vi "Temperature Warnings.vi"() -> ()   [LabVIEW 2018]
doc: "This VI is used to determine the string to output to the weather station based on the current temperature and limit settings.\n\nInputs: Current Temperature (DBL), Minimum Temperature (DBL), and Maximum Temperature (DBL).\nOutputs: Warning Text (string) and Warning? (Boolean)."
uses:
  Data.ctl
panel:
  out "Weather Data Out":T1={"Current Temperature"=0.0, "Max Temperature"=0.0, "Min Temperature"=0.0, "Warning?"=FALSE, "Warning Text"="No Warning", "Units"=enum."Celsius"}
  in  "Weather Data In":T1={"Current Temperature"=0.0, "Max Temperature"=0.0, "Min Temperature"=0.0, "Warning?"=FALSE, "Warning Text"="No Warning", "Units"=enum."Celsius"}
  out "Error Out":errorcluster
  in  "Error In":errorcluster
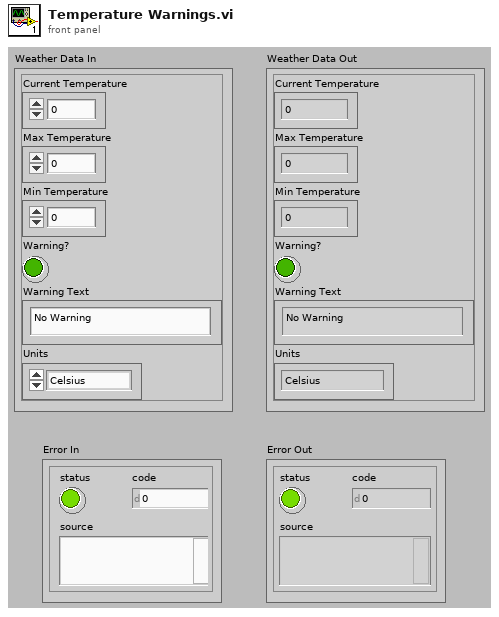
[diagram p1: front panel]
types:
  T1 = typedef "Data.ctl" = cluster{"Current Temperature":dbl, "Max Temperature":dbl, "Min Temperature":dbl, "Warning?":bool, "Warning Text":string, "Units":enum16{"Celsius", "Fahrenheit"}}
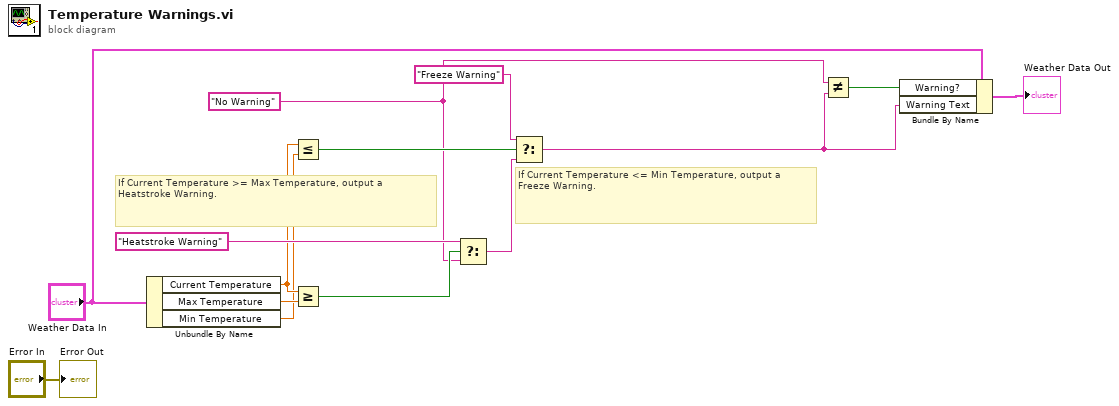
[diagram p0: block diagram]
diagram:
  w9 = "No Warning" ("f")
  # "If Current Temperature >= Max Temperature, output a Heatstroke Warning."
  # "If Current Temperature <= Min Temperature, output a Freeze Warning."
  n1 = Unbundle By Name("Weather Data In") -> ("Current Temperature"=w8:dbl, "Max Temperature"=w7:dbl, "Min Temperature"=w6:dbl)
  n2 = Less Or Equal?(x=w8, y=w6) -> (x <= y?=w11:bool)
  n3 = Greater Or Equal?(x=w8, y=w7) -> (x >= y?=w14:bool)
  n4 = Select(t="Heatstroke Warning", s=w14, f=w9) -> (s? t:f=w10:string)
  n5 = Select(t="Freeze Warning", s=w11, f=w10) -> (s? t:f=w2:string)
  n6 = Not Equal?(x=w9, y=w2) -> (x != y?=w1:bool)
  n7 = Bundle By Name(cluster="Weather Data In", "Warning?"=w1, "Warning Text"=w2) -> (→"Weather Data Out":T1)
  "Error Out" <- "Error In"
